vi "Generate Rectangle Sequence Images.vi"(6 "Predominant ROI type":T1=enum."Comp. volume", 7 "Imaging Protocol":T2=enum."Live Imaging", 8 "error in (no error)":errorcluster, 9 "Use connector pane path input":bool, 11 "TDMS file path & name":path) -> (0 "error out":errorcluster, 2 "Destination fiolder":path, 3 "tdms file to close":refnum<k34>)   [LabVIEW 2020]
uses:
  Typedefs/Imaging Protocols enum.ctl
  Typedefs/ROI ID Enum.ctl
  User Interface/Visualisation/Functional Imaging Viewer/SubVIs/Experiment header interface/Typedefs/Header file actions.ctl
  User Interface/Visualisation/Functional Imaging Viewer/SubVIs/Experiment header interface/Typedefs/Header file sections.ctl
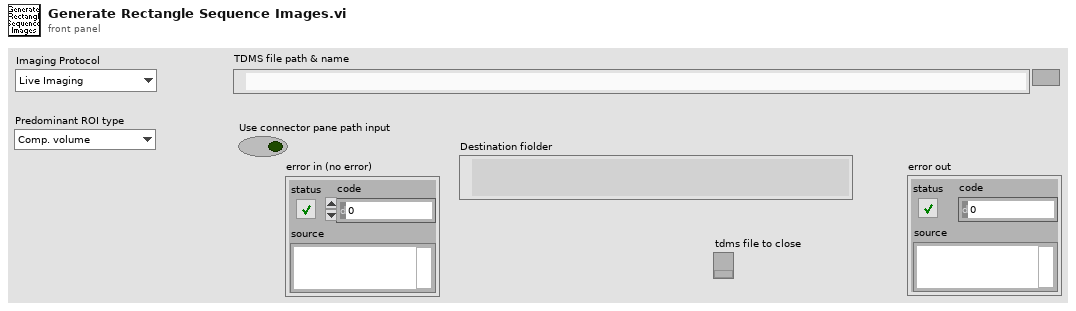
[diagram p1: front panel]
types:
  T1 = typedef "ROI ID Enum.ctl" = enum16{"Point", "MiniScan", "Comp. MiniScan", "Rectangle", "Comp. volume", "Arb. plane point", "None"}
  T2 = typedef "Imaging Protocols enum.ctl" = enum16{"AOL Z-Stack", "Motor Z Stack", "Functional Acquisition", "Single Plane Acquisition", "Volume Acquisition", "Live Imaging", "Live Plane Imaging", "Live Volume Imaging"}
  T3 = typedef "Header file sections.ctl" = enum16{"ALL SECTIONS", "LOGIN", "GLOBAL PARAMETERS", "CALIBRATION DATA", "IMAGING MODES", "TIME SERIES", "MOTOR Z-STACK", "AOL Z-STACK", "FUNCTIONAL IMAGING", "VOLUME IMAGING", "MOVEMENT CORRECTION", "CALIBRATION", "STATISTICS", "BIOLOGY INFORMATION"}
  T4 = typedef "Header file actions.ctl" = enum16{"Create", "Open", "Read All", "Read Section", "Write All", "Write Section", "Close"}
  T5 = typedef "Header parameters cluster-ALL.ctl" = cluster{"LOGIN":T6, "GLOBAL PARAMETERS":T7, "IMAGING MODES":T9, "TIME SERIES":T10, "MOTOR Z-STACK ":T13, "AOL Z-STACK":T14, "FUNCTIONAL IMAGING":T15, "VOLUME IMAGING":T15, "MOVEMENT CORRECTION":T19, "CALIBRATION":T21, "STATISTICS":T22, "BIOLOGY INFORMATION":T23, "Calibration Data":T24}
  T6 = typedef "Header params -Login.ctl" = cluster{"User":string, "Profile":string, "Software Version":string, "Experiment Date Time":timestamp}
  T7 = typedef "Header params-Global Parameters.ctl" = cluster{"MicroscopeID":string, "Microscope Type":string, "Objective":string, "Field of View (um)":dbl, "Fill time (us)":dbl, "Experiment Type":T8, "Stimuli Trigger":bool, "Speed Logging":bool}
  T8 = typedef "Experiment Type.ctl" = enum16{"In vivo", "In vitro", "Testing", "Calibration", "Other"}
  T9 = typedef "Header params-Imaging Modes.ctl" = cluster{"Time Series":bool, "Motor Zstack":bool, "AOL Zstack":bool, "Functional Imaging":bool, "Volume Imaging":bool}
  T10 = typedef "Header params-Time Series.ctl" = cluster{"Basic Image meta data":T11, "AOL z":dbl}
  T11 = typedef "Header params-Basic image meta data.ctl" = cluster{"Wavelength (nm)":dbl, "# averaged frames":dbl, "laser power (%)":dbl, "Pockels":dbl, "pixel dwell time (us)":dbl, "pmt 1":dbl, "pmt 2":dbl, "back apperture":dbl, "zoom":dbl, "field of view":dbl, "Frame Size":T12, "AOL x centre":dbl, "AOL y centre":dbl, "Stage x position":dbl, "Stage y position":dbl, "Stage z position":dbl}
  T12 = typedef "Frame Size.ctl" = u16
  T13 = typedef "Header params-Motor Z-stack.ctl" = cluster{"Hdr Basic Image meta data":T11, "Z Start":dbl, "Z Stop":dbl, "No of Planes":i32, "Laser Power (%) at Z Start":dbl, "Laser Power (%) at Z Stop":dbl}
  T14 = typedef "Header params-AOL Z-stack.ctl" = cluster{"Hdr Basic Image meta data":T11, "Z Start":dbl, "Z Stop":dbl, "No of Planes":i32, "Laser Power (%) at Z Start":dbl, "Laser Power (%) at Z Stop":dbl}
  T15 = typedef "Header params-Functional Imaging.ctl" = cluster{"Functional Mode":T16, "Variable Length":bool, "Variable Resolution":bool, "Pockels Modulation":bool, "Stimuli Trigger":bool, "Cool down enabled":bool, "AOL Mode":T17, "Plane Mode":T18, "Miniscan Dwell time per pixel (us)":dbl, "poi dwell time":dbl, "Number of trials":dbl, "Number of cycles":dbl, "Number of pois":dbl, "Number of miniscans":dbl, "Number of pixels in miniscan":dbl, "Rectangle ROI length":dbl, "Rectangle ROI height":dbl, "Frame rate (fps)":dbl, "Acquisition Length":dbl, "video length (sec)":dbl, "Stimuli delay (sec)":dbl, "Cool down time (sec)":dbl, "Basic Image meta data":T11, "Z Start (um)":dbl, "Z Stop (um)":dbl}
  T16 = typedef "Functional Mode.ctl" = enum16{"Point", "Line", "Patch", "Plane", "Volume"}
  T17 = typedef "AOL modes.ctl" = enum16{"Raster", "Structural", "Pointing", "Mini Scan", "Alignment"}
  T18 = typedef "Plane Mode.ctl" = u16
  T19 = typedef "Header params-Movement correction.ctl" = cluster{"Movement Correction":bool, "Axial Reference":bool, "Reference Source":T20, "Full Frame Size":dbl, "Reference Field of View":dbl, "Reference Zoom":dbl, "Reference dwell time (us)":dbl, "Reference X Pixels":dbl, "Reference Y Pixels":dbl, "Number of Z lines":dbl, "Size of Z pixels":dbl, "Axial Pixels":dbl, "Ignore Z lines":dbl, "Reference Scan Cycles":dbl, "Reference Threshold XY":dbl, "Reference Threshold Z":dbl, "Reference Average XY":dbl, "Reference Average Z":dbl, "Proportional Scale":dbl, "Integral Scale":dbl, "Proportional Scale Z":dbl, "Integral Scale Z":dbl, "Diff Threshold":dbl, "Diff Threshold Z":dbl, "Sliding Average":bool, "Reference count reset enabled":bool, "Scan Interval (ms)":dbl, "Ref Plot Refresh Rate (ms)":dbl}
  T20 = typedef "Reference source.ctl" = enum16{"Green channel", "Red channel"}
  T21 = typedef "Header params-Calibration Setup.ctl" = cluster{"Pockels Calibration File":path, "Calibration_ini file":path, "Setup_ini file":path}
  T22 = typedef "Header params-statistics.ctl" = cluster{"Z-stack duration (sec)":dbl, "Number of acquired data-points":dbl, "Acquisition time (ms)":dbl, "Number of acquired frames":dbl, "Intertrial times":dbl[]}
  T23 = typedef "Biology Information.ctl" = cluster{"Animal Code or Name":string, "Animal DoB":string, "Animal Age":string, "Animal Sex":string, "Animal Weight":string, "Date of Injection":string, "Date of Implant":string, "Site of Injection":string, "Animal Ear Notch":string, "AAV constructs":string, "Genetic background":string, "Optical reporter":string, "Region of brain imaged":string, "Other \ncomments":string}
  T24 = typedef "Header params-calibration data.ctl" = cluster{"Objective Name":string, "Calibration Wavelength":dbl, "Sum X":dbl, "Sum Y":dbl, "Diff X":dbl, "Diff Y":dbl, "Distortion Correction":dbl, " Z norm to um Scaling":dbl, " X norm to um Scaling":dbl}
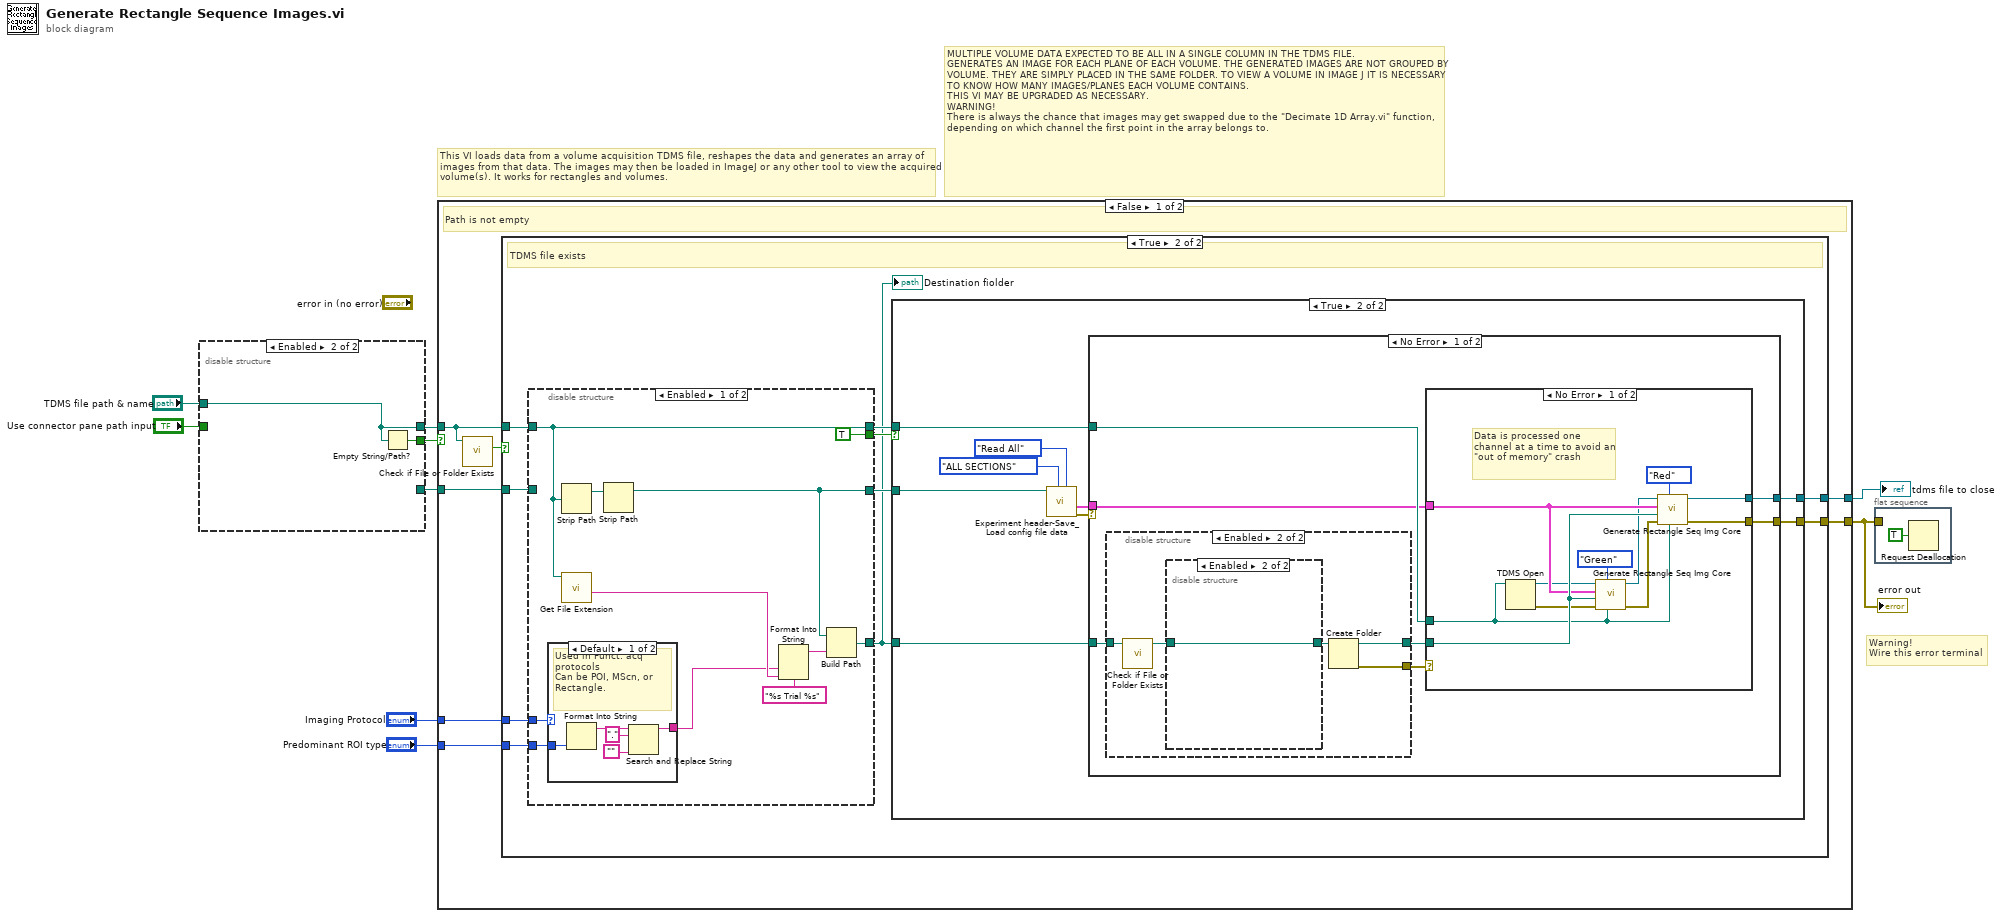
[diagram p0: block diagram]
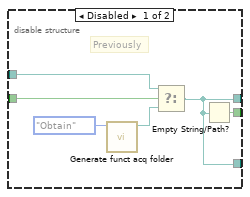
[diagram p2: hidden frame]
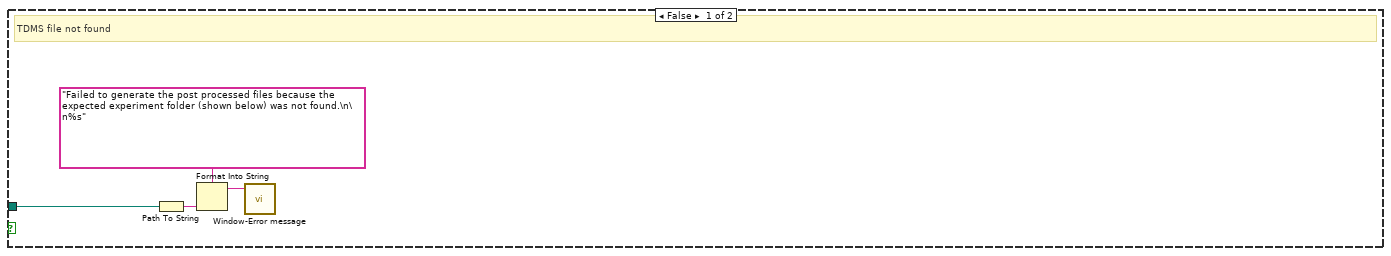
[diagram p3: hidden frame]
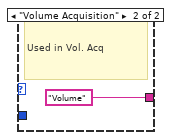
[diagram p4: hidden frame]
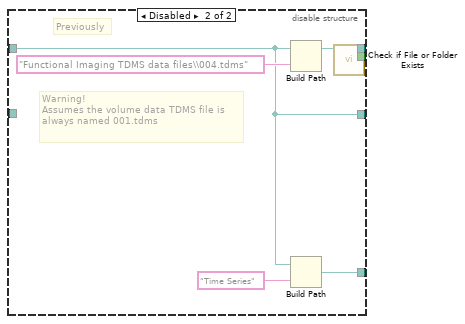
[diagram p5: hidden frame]
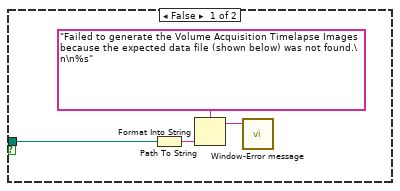
[diagram p6: hidden frame]
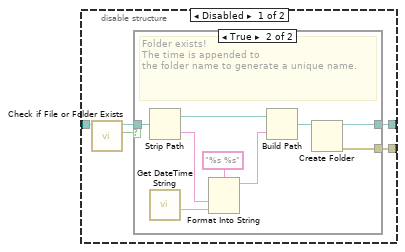
[diagram p7: hidden frame]
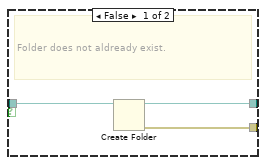
[diagram p8: hidden frame]
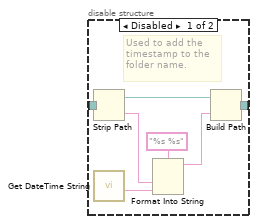
[diagram p9: hidden frame]
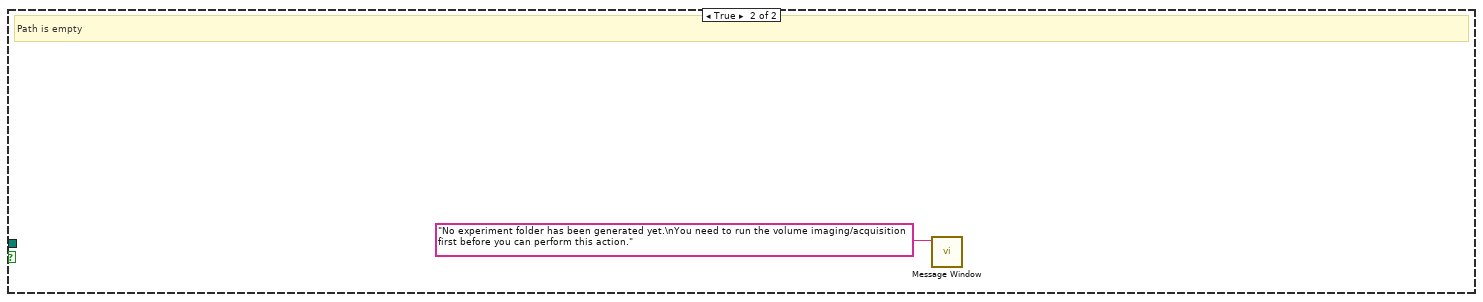
[diagram p12: hidden frame]
diagram:
  # "This VI loads data from a volume acquisition TDMS file, reshapes the data and generates an array of images from that data. The images may then be loaded in ImageJ or any other tool to view the acquired volume(s). It works for rectangles and volumes."
  # "Warning!\nWire this error terminal"
  # "MULTIPLE VOLUME DATA EXPECTED TO BE ALL IN A SINGLE COLUMN IN THE TDMS FILE.\nGENERATES AN IMAGE FOR EACH PLANE OF EACH VOLUME. THE GENERATED IMAGES ARE NOT GROUPED BY VOLUME. THEY ARE SIMPLY PLACED IN THE SAME FOLDER. TO VIEW A VOLUME IN IMAGE J IT IS NECESSARY TO KNOW HOW MANY IMAGES/PLANES EACH VOLUME CONTAINS.\nTHIS VI MAY BE UPGRADED AS NECESSARY.\nWARNING!\nThere is always the chance that images may get swapped due to the \"Decimate 1D Array.vi\" function, depending on which channel the first point in the array belongs to."
  n1 = disable-structure shown="Enabled" {
    disable-tunnel: [w14 w17] -> w9
    disable-tunnel: [w10 w16] -> w8
    disable-tunnel: "TDMS file path & name" -> [w13 w16]
    disable-tunnel: "Use connector pane path input" -> [w12 _]
    disable-tunnel: [w10 _] -> w5
    frame Disabled {
      # "Previously"
      n2 = call "Generate funct acq folder.vi"("Function"=enum16{"Generate", "Obtain"}."Obtain") -> ("Funct acq experiment folder path"=w11:path)  [unwired: 9 in, 1 out]
      n3 = Select(t=w13, s=w12, f=w11) -> (s? t:f=w10:path)
      n4 = Empty String/Path?(string/path=w10) -> (empty?=w14:bool)
    }
    frame Enabled {
      n5 = Empty String/Path?(string/path=w16) -> (empty?=w17:bool)
    }
  }
  n6 = case shown="False" w9 {
    tunnel: w8 -> [w23 _]
    tunnel: w5 -> [w22 _]
    tunnel: [w21 _] -> w2
    tunnel: "Imaging Protocol" -> [w20 _]
    tunnel: "Predominant ROI type" -> [w19 _]
    tunnel: [w18 _] -> w1
    frame False {
      # "Path is not empty"
      n7 = call <vilib>:"Check if File or Folder Exists.vi"("path"=w23) -> ("file or folder exists?"=w24:bool)  [unwired: 8 in, 2 out]
      n8 = case shown="True" w24 {
        tunnel: w23 -> [w27 w35]
        tunnel: w22 -> [_ w36]
        tunnel: [_ w33] -> w21
        tunnel: w20 -> [_ w31]
        tunnel: w19 -> [_ w30]
        tunnel: [_ w29] -> w18
        frame False {
          # "TDMS file not found"
          n9 = Path To String(path=w27) -> (string=w26:string)
          n10 = Format Into String(format string="Failed to generate the post processed files because the expected experiment folder (shown below) was not found.\n\n%s", w26) -> (resulting string=w25:string)  [unwired: 2 in, 1 out]
          n11 = call "Window-Error message.vi"("Message"=w25) -> ()  [unwired: 10 in, 1 out]
        }
        frame True {
          # "TDMS file exists"
          n12 = disable-structure shown="Enabled" {
            disable-tunnel: [TRUE ("file or folder exists?") w62] -> w38
            disable-tunnel: [w43 w61] -> w37
            disable-tunnel: [w49 w57] -> w32
            disable-tunnel: w35 -> [w43 w56]
            disable-tunnel: w36 -> [_ _]
            disable-tunnel: [w46 w56] -> w34
            disable-tunnel: w31 -> [w45 _]
            disable-tunnel: w30 -> [w44 _]
            frame Enabled {
              n13 = case shown="Default" w45 {
                tunnel: w44 -> [w54 _]
                tunnel: [w50 "Volume" ("result string")] -> w40
                frame Default {
                  # "Used in Funct. acq protocols\nCan be POI, MScn, or Rectangle."
                  n14 = Format Into String(w54) -> (resulting string=w53:string)  [unwired: 3 in, 1 out]
                  n15 = Search and Replace String(input string=w53, search string=".", replace string="" ("replace string (\"\")")) -> (result string=w50:string)  [unwired: 5 in, 3 out]
                }
                frame "Volume Acquisition" {
                  # "Used in Vol. Acq"
                }
              }
              n16 = Strip Path(path=w43) -> (stripped path=w48:path)  [unwired: 1 out]
              n17 = call <vilib>:"Get File Extension.vi"("file"=w43) -> ("filename without extension"=w41:string)  [unwired: 6 in, 4 out]
              n18 = Strip Path(path=w48) -> (stripped path=w46:path)  [unwired: 1 out]
              n19 = Format Into String(format string="%s Trial %s", w40, w41) -> (resulting string=w39:string)  [unwired: 2 in, 1 out]
              n20 = Build Path(base path=w46, name or relative path=w39) -> (appended path=w49:path)
            }
            frame Disabled {
              # "Previously"
              # "Warning!\nAssumes the volume data TDMS file is always named 001.tdms"
              n21 = Build Path(base path=w56, name or relative path="Functional Imaging TDMS data files\\004.tdms") -> (appended path=w60:path)
              n22 = Build Path(base path=w56, name or relative path="Time Series") -> (appended path=w57:path)
              n23 = call <vilib>:"Check if File or Folder Exists.vi"("path"=w60) -> ("file or folder exists?"=w62:bool, "dup path"=w61:path)  [unwired: 8 in, 1 out]
            }
          }
          "Destination fiolder" <- w32
          n24 = case shown="True" w38 {
            tunnel: w32 -> [_ w75]
            tunnel: w34 -> [_ w72]
            tunnel: w37 -> [w63 w74]
            tunnel: [_ w70] -> w33
            tunnel: [_ w69] -> w29
            frame False {
              n25 = Path To String(path=w63) -> (string=w64:string)
              n26 = Format Into String(format string="Failed to generate the Volume Acquisition Timelapse Images because the expected data file (shown below) was not found.\n\n%s", w64) -> (resulting string=w65:string)  [unwired: 2 in, 1 out]
              n27 = call "Window-Error message.vi"("Message"=w65) -> ()  [unwired: 10 in, 1 out]
            }
            frame True {
              n28 = call "Experiment header-Save_Load config file data.vi"("Header file actions"=Header_file_actions."Read All", "Header file sections"=Header_file_sections."ALL SECTIONS", "Experiment data folder path"=w72) -> ("error out"=w71:errorcluster, "All header parameters out"=w73:T5)  [unwired: 7 in]
              n29 = case shown="No Error" w71 {
                tunnel: w75 -> [w82 _]
                tunnel: w74 -> [w81 _]
                tunnel: w73 -> [w77 _]
                tunnel: [w78 _] -> w70
                tunnel: [w76 _] -> w69
                frame No Error {
                  n30 = disable-structure shown="Enabled" {
                    disable-tunnel: w82 -> [w87 w104]
                    disable-tunnel: [w84 w102] -> w80
                    disable-tunnel: [w83 w101] -> w79
                    frame Disabled {
                      n31 = call <vilib>:"Check if File or Folder Exists.vi"("path"=w87) -> ("file or folder exists?"=w85:bool, "dup path"=w86:path)  [unwired: 8 in, 1 out]
                      n32 = case shown="True" w85 {
                        tunnel: [w90 w92] -> w83
                        tunnel: [w89 w91] -> w84
                        tunnel: w86 -> [w88 w98]
                        frame False {
                          # "Folder does not aldready exist."
                          n33 = Create Folder(path (use dialog)=w88) -> (created path=w90:path, error out=w89:errorcluster)  [unwired: 2 in, 1 out]
                        }
                        frame True {
                          # "Folder exists!\nThe time is appended to\nthe folder name to generate a unique name."
                          n34 = Strip Path(path=w98) -> (stripped path=w99:path, name=w97:string)
                          n35 = call <userlib>:"Get DateTime String.vi"() -> ("Time string"=w96:string)  [unwired: 10 in, 1 out]
                          n36 = Format Into String(format string="%s %s", w97, w96) -> (resulting string=w94:string)  [unwired: 2 in, 1 out]
                          n37 = Build Path(base path=w99, name or relative path=w94) -> (appended path=w93:path)
                          n38 = Create Folder(path (use dialog)=w93) -> (created path=w92:path, error out=w91:errorcluster)  [unwired: 2 in, 1 out]
                        }
                      }
                    }
                    frame Enabled {
                      n39 = call <vilib>:"Check if File or Folder Exists.vi"("path"=w104) -> ("dup path"=w103:path)  [unwired: 8 in, 2 out]
                      n40 = disable-structure shown="Enabled" {
                        disable-tunnel: w103 -> [w111 w112]
                        disable-tunnel: [w105 w112] -> w100
                        frame Disabled {
                          # "Used to add the \ntimestamp to the \nfolder name."
                          n41 = Strip Path(path=w111) -> (stripped path=w110:path, name=w109:string)
                          n42 = call <userlib>:"Get DateTime String.vi"() -> ("Time string"=w108:string)  [unwired: 10 in, 1 out]
                          n43 = Format Into String(format string="%s %s", w109, w108) -> (resulting string=w106:string)  [unwired: 2 in, 1 out]
                          n44 = Build Path(base path=w110, name or relative path=w106) -> (appended path=w105:path)
                        }
                        frame Enabled {
                        }
                      }
                      n45 = Create Folder(path (use dialog)=w100) -> (created path=w101:path, error out=w102:errorcluster)  [unwired: 2 in, 1 out]
                    }
                  }
                  n46 = case shown="No Error" w80 {
                    selector: w80 -> [_ w124]
                    tunnel: w79 -> [w123 _]
                    tunnel: w81 -> [w115 _]
                    tunnel: w77 -> [w122 _]
                    tunnel: [w114 w124] -> w78
                    tunnel: [w113 _] -> w76
                    frame No Error {
                      # "Data is processed one channel at a time to avoid an \"out of memory\" crash"
                      n47 = TDMS Open(11:w115) -> (0:w117:errorcluster, 3:w116:refnum<k34>)  [unwired: 6 in]
                      n48 = call "Generate Rectangle Seq Img Core.vi"("TDMS file path & name"=w115, "Channel to process"=enum16{"Red", "Green"}."Green", "error in (no error)"=w117, "<Vol images/video folder>"=w123, "All header parameters"=w122, "tdms file ref"=w116) -> ("error out"=w121:errorcluster, "tdms file out"=w118:refnum<k34>)  [unwired: 4 in]
                      n49 = call "Generate Rectangle Seq Img Core.vi"("TDMS file path & name"=w115, "Channel to process"=enum16{"Red", "Green"}."Red", "error in (no error)"=w121, "<Vol images/video folder>"=w123, "All header parameters"=w122, "tdms file ref"=w118) -> ("error out"=w114:errorcluster, "tdms file out"=w113:refnum<k34>)  [unwired: 4 in]
                    }
                    frame Error {
                    }
                  }
                }
                frame Error {
                  # "Error reporting handled inside the subVI."
                }
              }
            }
          }
        }
      }
    }
    frame True {
      # "Path is empty"
      n50 = call "Message Window.vi"("Message string"="No experiment folder has been generated yet.\nYou need to run the volume imaging/acquisition first before you can perform this action.") -> ()  [unwired: 10 in, 1 out]
    }
  }
  "error out" <- w2
  "tdms file to close" <- w1
  n51 = flat-sequence {
    tunnel: w2 -> [_]
    frame #0 {
      n52 = Request Deallocation(TRUE ("flag")) -> ()
    }
  }
